vi "myCommOut_visa.vi"(0 "VISA资源名称":refnum<visa-resource-name>, 1 "freqs rows":i32[][](array[numeric]), 2 "log输入":string, 3 "默认幅值 Amp0":u8(ring)=2 items=["10.0", "5.0", "1.0", "0.5", "0.1", "0.05", "0.01"], 5 "实际幅值 Amp":u8(ring)=1 items=["= Amp0", "= Amp0 / freq"], 7 "t_wait":dbl=0.04, 9 "扰动注入模式":i32(ring) items=["无注入", "单相注入", "d轴注入", "q轴注入", "正(负)序注入"], 10 "最大同时扫频数":u32=5 min=1 max=10, 11 "错误输入（无错误）":errorcluster, 12 "基波频率":u32=50, 14 "存在DSP":bool) -> (4 "VISA资源名称 2":refnum<visa-resource-name>, 8 "error out":bool, 13 "log输出":string, 15 "错误输出":errorcluster)   [LabVIEW 2024]
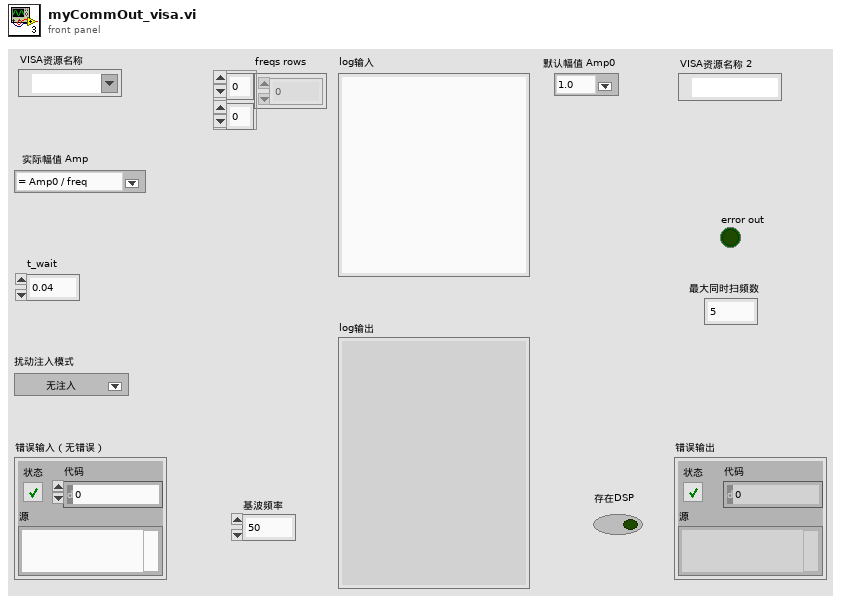
[diagram p1: front panel]
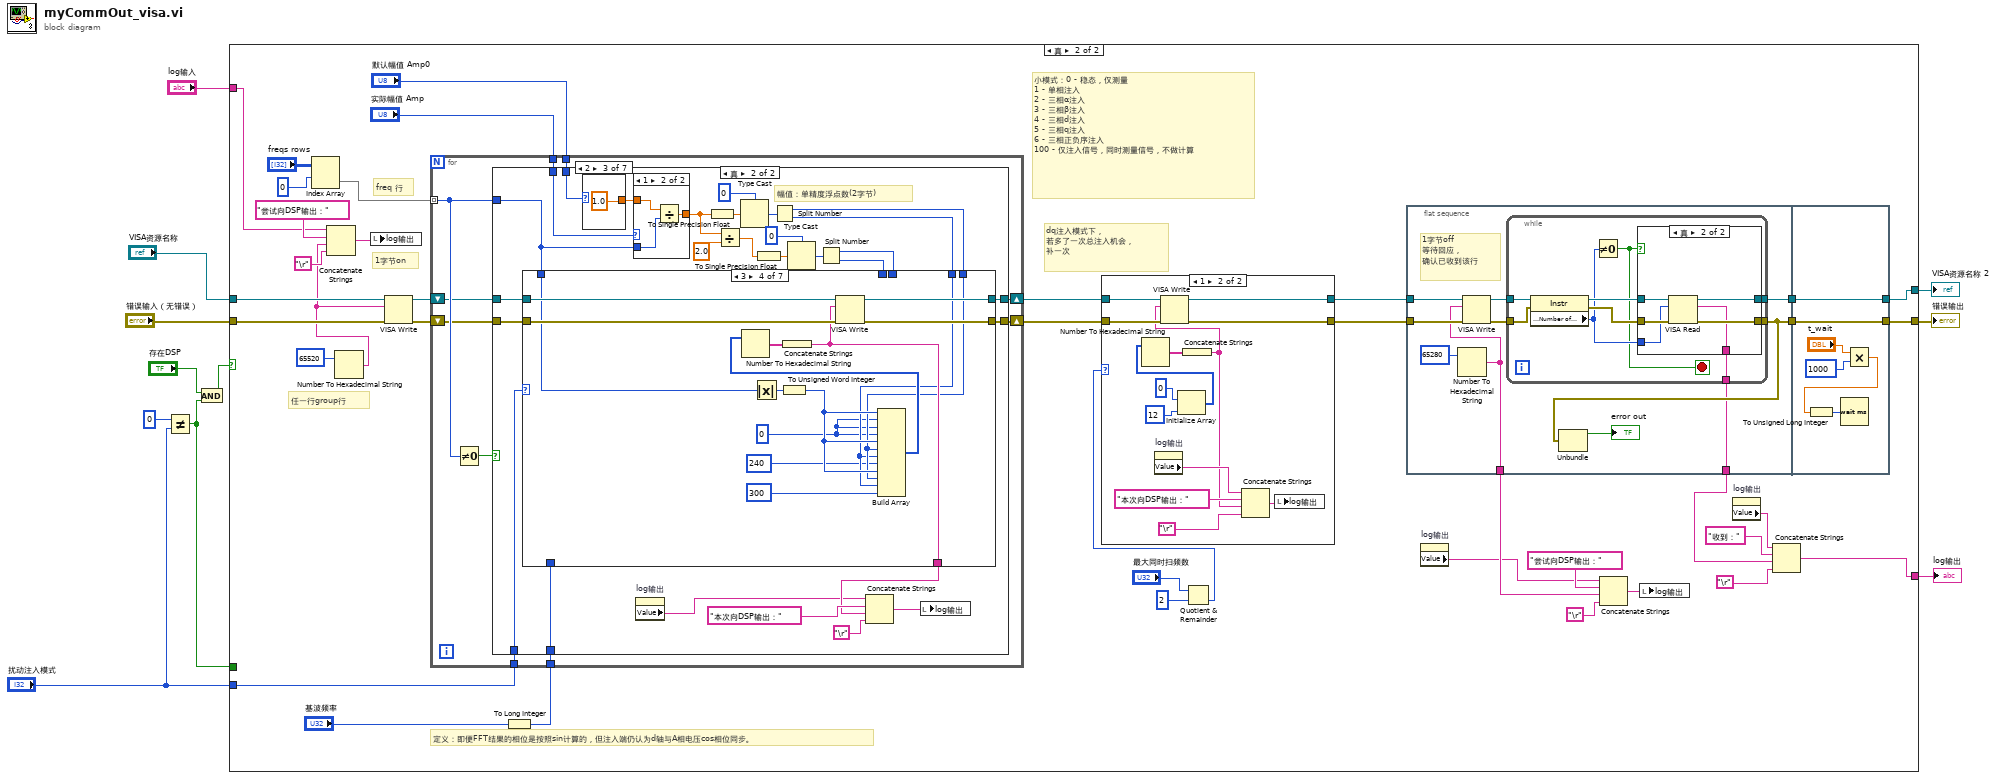
[diagram p0: block diagram]
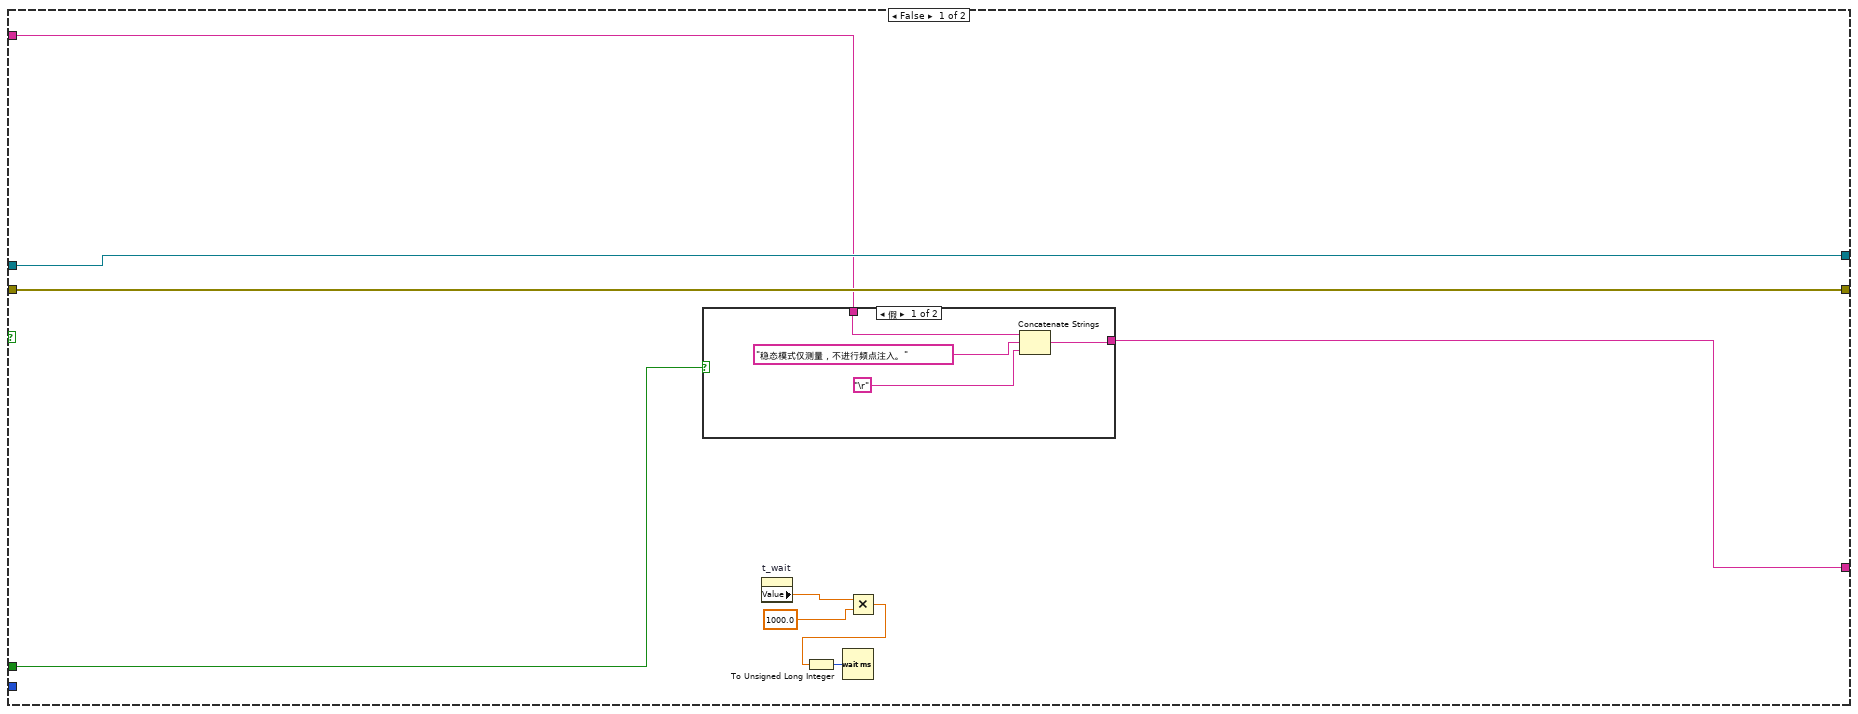
[diagram p2: hidden frame]
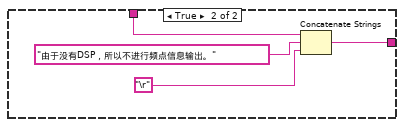
[diagram p3: hidden frame]
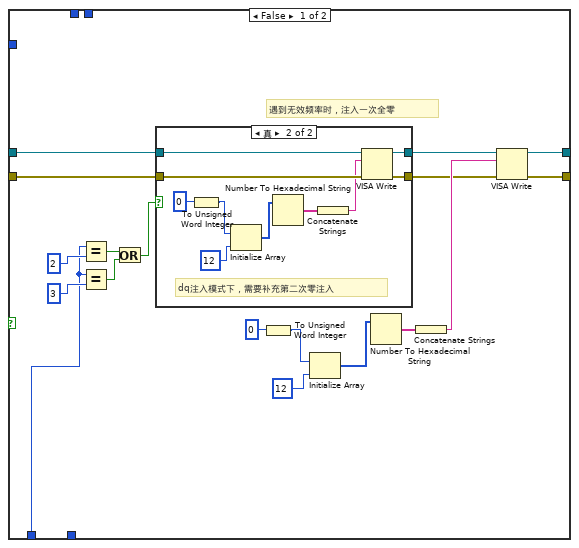
[diagram p6: hidden frame]
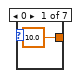
[diagram p9: hidden frame]
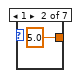
[diagram p10: hidden frame]
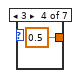
[diagram p11: hidden frame]
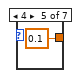
[diagram p12: hidden frame]
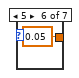
[diagram p13: hidden frame]
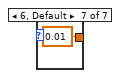
[diagram p14: hidden frame]
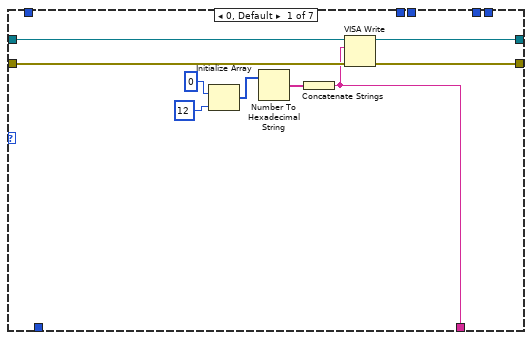
[diagram p15: hidden frame]
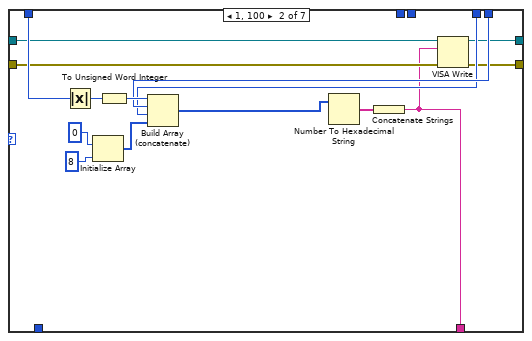
[diagram p16: hidden frame]
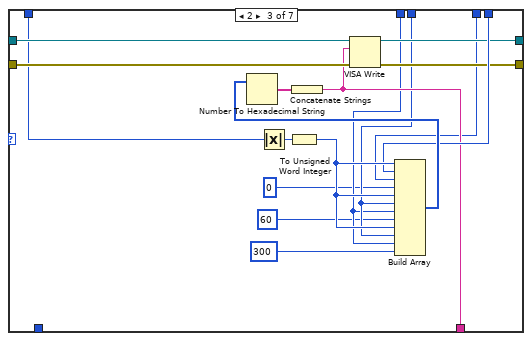
[diagram p17: hidden frame]
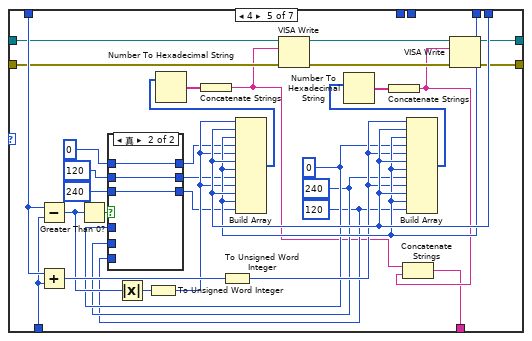
[diagram p18: hidden frame]
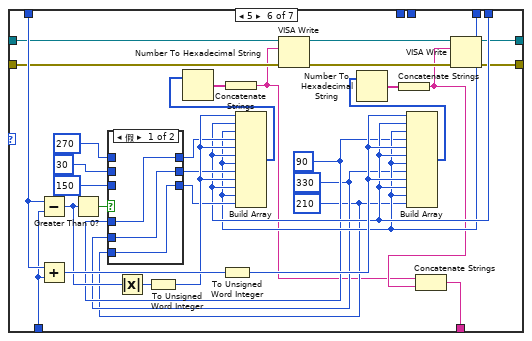
[diagram p20: hidden frame]
diagram:
  n1 = Not Equal?(x=0, y="扰动注入模式") -> (x != y?=w3:bool)
  n2 = And(x="存在DSP", y=w3) -> (x .and. y?=w4:bool)
  n3 = case shown="真" w4 {
    tunnel: "VISA资源名称" -> [w20 w54]
    tunnel: "错误输入（无错误）" -> [w19 w53]
    tunnel: [w20 w49] -> w9
    tunnel: [w19 w48] -> w8
    tunnel: "log输入" -> [w15 w43]
    tunnel: [w14 w38] -> w6
    tunnel: "扰动注入模式" -> [_ w29]
    tunnel: w3 -> [w12 _]
    frame False {
      n4 = case shown="假" w12 {
        tunnel: w15 -> [w21 w26]
        tunnel: [w22 w25] -> w14
        frame False {
          n5 = Concatenate Strings(w21, "稳态模式仅测量，不进行频点注入。", "\r") -> (w22:string)
        }
        frame True {
          n6 = Concatenate Strings(w26, "由于没有DSP，所以不进行频点信息输出。", "\r") -> (w25:string)
        }
      }
      n7 = property on="t_wait" class="DigNum (严格)"() -> ("Value"=w13:dbl)  [unwired: 2 in, 2 out]
      n8 = Multiply(x=w13, y=1000.0) -> (x*y=w18:dbl)
      n9 = To Unsigned Long Integer(number=w18) -> (unsigned 32bit integer=w17:u32)
      n10 = Wait (ms)(milliseconds to wait=w17) -> ()  [unwired: 1 out]
    }
    frame True {
      # "小模式：0 - 稳态，仅测量\n1 - 单相注入\n2 - 三相α注入\n3 - 三相β注入\n4 - 三相d注入\n5 - 三相q注入\n6 - 三相正负序注入\n100 - 仅注入信号，同时测量信号，不做计算"
      # "freq 行"
      # "dq注入模式下，\n若多了一次总注入机会，\n补一次"
      # "任一行group行"
      # "1字节on"
      # "定义：即便FFT结果的相位是按照sin计算的，但注入端仍认为d轴与A相电压cos相位同步。"
      n11 = Index Array(array="freqs rows", index (row)=0 ("索引")) -> (element=w31:i32[])  [unwired: 1 in]
      n12 = Number To Hexadecimal String(2:u16 65520) -> (0:w45:string)  [unwired: 1 in]
      n13 = Concatenate Strings(w43, "尝试向DSP输出：", w45, "\r") -> (w44:string)
      n14 = local write "log输出"(w44) -> ()
      n15 = VISA Write(VISA resource name=w54, write buffer=w45, error in (no error)=w53) -> (VISA resource name out=w62:refnum<visa-resource-name>, error out=w63:errorcluster)  [unwired: 1 out]
      n16 = To Long Integer(number="基波频率") -> (32bit integer=w55:i32)
      n17 = for {
        shift-right: [w121] -> w60
        shift-left: w62 -> [w123]
        shift-right: [w120] -> w59
        shift-left: w63 -> [w122]
        tunnel: w31 -> [w125] mode=indexing
        tunnel: w29 -> [w119]
        tunnel: "实际幅值 Amp" -> [w118]
        tunnel: "默认幅值 Amp0" -> [w117]
        tunnel: w55 -> [w116]
        n18 = Not Equal To 0?(x=w125) -> (x != 0?=w124:bool)
        n19 = case shown="真" w124 {
          tunnel: w125 -> [_ w169]
          tunnel: [w127 w174] -> w120
          tunnel: w123 -> [w139 w177]
          tunnel: [w128 w175] -> w121
          tunnel: w122 -> [w140 w176]
          tunnel: w119 -> [w133 w173]
          tunnel: w118 -> [_ w172]
          tunnel: w117 -> [_ w171]
          tunnel: w116 -> [_ w170]
          frame False {
            # "遇到无效频率时，注入一次全零"
            n20 = Equal?(x=w133, y=2) -> (x = y?=w135:bool)
            n21 = Equal?(x=w133, y=3) -> (x = y?=w136:bool)
            n22 = Or(x=w135, y=w136) -> (x .or. y?=w134:bool)
            n23 = case shown="真" w134 {
              tunnel: w140 -> [w144 w151]
              tunnel: w139 -> [w145 w152]
              tunnel: [w145 w146] -> w129
              tunnel: [w144 w147] -> w126
              frame False {
              }
              frame True {
                # "dq注入模式下，需要补充第二次零注入"
                n24 = To Unsigned Word Integer(number=u16 0) -> (unsigned 16bit integer=w154:u16)
                n25 = Initialize Array(w154, 12 ("维数大小")) -> (w149:u16[])
                n26 = Number To Hexadecimal String(2:w149) -> (0:w150:string[])  [unwired: 1 in]
                n27 = Concatenate Strings(w150) -> (w148:string)
                n28 = VISA Write(VISA resource name=w152, write buffer=w148, error in (no error)=w151) -> (VISA resource name out=w146:refnum<visa-resource-name>, error out=w147:errorcluster)  [unwired: 1 out]
              }
            }
            n29 = To Unsigned Word Integer(number=u16 0) -> (unsigned 16bit integer=w142:u16)
            n30 = Initialize Array(w142, 12 ("维数大小")) -> (w131:u16[])
            n31 = Number To Hexadecimal String(2:w131) -> (0:w132:string[])  [unwired: 1 in]
            n32 = Concatenate Strings(w132) -> (w130:string)
            n33 = VISA Write(VISA resource name=w129, write buffer=w130, error in (no error)=w126) -> (VISA resource name out=w128:refnum<visa-resource-name>, error out=w127:errorcluster)  [unwired: 1 out]
          }
          frame True {
            # "幅值：单精度浮点数(2字节)"
            n34 = case shown="2" w171 {
              tunnel: [10.0 5.0 1.0 0.5 0.1 0.05 0.01] -> w183
              frame 0 {
              }
              frame 1 {
              }
              frame 2 {
              }
              frame 3 {
              }
              frame 4 {
              }
              frame 5 {
              }
              frame 6, Default {
              }
            }
            n35 = case shown="1" w172 {
              tunnel: w183 -> [w184 w187]
              tunnel: w169 -> [_ w186]
              tunnel: [w184 w185] -> w163
              frame 0, Default {
              }
              frame 1 {
                n36 = Divide(x=w187, y=w186) -> (x/y=w185:dbl)
              }
            }
            n37 = property on="log输出" class="Str"() -> ("Value"=w165:string)  [unwired: 2 in, 2 out]
            n38 = To Single Precision Float(number=w163) -> (single precision float=w182:sgl)
            n39 = Divide(x=w163, y=2.0) -> (x/y=w159:dbl)
            n40 = Type Cast(type=0, x=w182) -> (*(type *) &x=w180:i32)
            n41 = To Single Precision Float(number=w159) -> (single precision float=w161:sgl)
            n42 = Split Number(x=w180) -> (hi(x)=w179:u16, lo(x)=w178:u16)
            n43 = Type Cast(type=0, x=w161) -> (*(type *) &x=w156:i32)
            n44 = Split Number(x=w156) -> (hi(x)=w158:u16, lo(x)=w157:u16)
            n45 = case shown="3" w173 {
              tunnel: w169 -> [_ w217 w228 w244 w279 w311 w340]
              tunnel: w179 -> [_ w213 w229 w240 w281 w310 w339]
              tunnel: w178 -> [_ w212 w224 w239 w280 w309 w338]
              tunnel: [w200 w209 w225 w241 w257 w296 w332] -> w175
              tunnel: w177 -> [w197 w210 w231 w246 w262 w298 w335]
              tunnel: [w199 w207 w226 w242 w258 w295 w333] -> w174
              tunnel: w176 -> [w198 w208 w230 w245 w261 w297 w334]
              tunnel: w170 -> [_ _ _ _ w264 w302 _]
              tunnel: [w195 w204 w227 w243 w251 w289 w330] -> w166
              tunnel: w158 -> [_ _ w223 _ _ _ _]
              tunnel: w157 -> [_ _ w222 _ _ _ _]
              frame 0, Default {
                n46 = Initialize Array(u16 0, 12 ("维数大小")) -> (w196:u16[])
                n47 = Number To Hexadecimal String(2:w196) -> (0:w201:string[])  [unwired: 1 in]
                n48 = Concatenate Strings(w201) -> (w195:string)
                n49 = VISA Write(VISA resource name=w197, write buffer=w195, error in (no error)=w198) -> (VISA resource name out=w200:refnum<visa-resource-name>, error out=w199:errorcluster)  [unwired: 1 out]
              }
              frame 1, 100 {
                n50 = Absolute Value(x=w217) -> (abs(x)=w218:i32)
                n51 = Initialize Array(u16 0, 8 ("维数大小")) -> (w206:u16[])
                n52 = To Unsigned Word Integer(number=w218) -> (unsigned 16bit integer=w214:u16)
                n53 = Build Array (concatenate)(w214, w213, w212, w206) -> (w205:u16[])
                n54 = Number To Hexadecimal String(2:w205) -> (0:w211:string[])  [unwired: 1 in]
                n55 = Concatenate Strings(w211) -> (w204:string)
                n56 = VISA Write(VISA resource name=w210, write buffer=w204, error in (no error)=w208) -> (VISA resource name out=w209:refnum<visa-resource-name>, error out=w207:errorcluster)  [unwired: 1 out]
              }
              frame 2 {
                n57 = Absolute Value(x=w228) -> (abs(x)=w235:i32)
                n58 = To Unsigned Word Integer(number=w235) -> (unsigned 16bit integer=w234:u16)
                n59 = Build Array(w234, w229, w224, u16 0, w234, w223, w222, u16 60, w234, w223, w222, u16 300) -> (w232:u16[])
                n60 = Number To Hexadecimal String(2:w232) -> (0:w233:string[])  [unwired: 1 in]
                n61 = Concatenate Strings(w233) -> (w227:string)
                n62 = VISA Write(VISA resource name=w231, write buffer=w227, error in (no error)=w230) -> (VISA resource name out=w225:refnum<visa-resource-name>, error out=w226:errorcluster)  [unwired: 1 out]
              }
              frame 3 {
                w238 = u16 0
                n63 = Absolute Value(x=w244) -> (abs(x)=w250:i32)
                n64 = To Unsigned Word Integer(number=w250) -> (unsigned 16bit integer=w249:u16)
                n65 = Build Array(w249, w238, w238, w238, w249, w240, w239, u16 240, w249, w240, w239, u16 300) -> (w247:u16[])
                n66 = Number To Hexadecimal String(2:w247) -> (0:w248:string[])  [unwired: 1 in]
                n67 = Concatenate Strings(w248) -> (w243:string)
                n68 = VISA Write(VISA resource name=w246, write buffer=w243, error in (no error)=w245) -> (VISA resource name out=w241:refnum<visa-resource-name>, error out=w242:errorcluster)  [unwired: 1 out]
              }
              frame 4 {
                w265 = u16 120
                w266 = u16 240
                w267 = u16 0
                n69 = Subtract(x=w279, y=w264) -> (x-y=w276:i32)
                n70 = Add(x=w279, y=w264) -> (x+y=w278:i32)
                n71 = Greater Than 0?(x=w276) -> (x > 0?=w274:bool)
                n72 = case shown="真" w274 {
                  tunnel: u16 0 -> [_ w288]
                  tunnel: u16 120 -> [_ w287]
                  tunnel: u16 240 -> [_ w286]
                  tunnel: [w283 w288] -> w270
                  tunnel: [w284 w287] -> w269
                  tunnel: [w285 w286] -> w268
                  tunnel: w267 -> [w283 _]
                  tunnel: w266 -> [w284 _]
                  tunnel: w265 -> [w285 _]
                  frame False {
                  }
                  frame True {
                  }
                }
                n73 = Absolute Value(x=w276) -> (abs(x)=w282:i32)
                n74 = To Unsigned Word Integer(number=w282) -> (unsigned 16bit integer=w275:u16)
                n75 = To Unsigned Word Integer(number=w278) -> (unsigned 16bit integer=w277:u16)
                n76 = Build Array(w275, w281, w280, w270, w275, w281, w280, w269, w275, w281, w280, w268) -> (w254:u16[])
                n77 = Number To Hexadecimal String(2:w254) -> (0:w255:string[])  [unwired: 1 in]
                n78 = Concatenate Strings(w255) -> (w253:string)
                n79 = VISA Write(VISA resource name=w262, write buffer=w253, error in (no error)=w261) -> (VISA resource name out=w260:refnum<visa-resource-name>, error out=w259:errorcluster)  [unwired: 1 out]
                n80 = Build Array(w277, w281, w280, w267, w277, w281, w280, w266, w277, w281, w280, w265) -> (w256:u16[])
                n81 = Number To Hexadecimal String(2:w256) -> (0:w263:string[])  [unwired: 1 in]
                n82 = Concatenate Strings(w263) -> (w252:string)
                n83 = Concatenate Strings(w253, w252) -> (w251:string)
                n84 = VISA Write(VISA resource name=w260, write buffer=w252, error in (no error)=w259) -> (VISA resource name out=w257:refnum<visa-resource-name>, error out=w258:errorcluster)  [unwired: 1 out]
              }
              frame 5 {
                w306 = u16 210
                w307 = u16 330
                w308 = u16 90
                n85 = Subtract(x=w311, y=w302) -> (x-y=w317:i32)
                n86 = Add(x=w311, y=w302) -> (x+y=w319:i32)
                n87 = Greater Than 0?(x=w317) -> (x > 0?=w315:bool)
                n88 = case shown="假" w315 {
                  tunnel: u16 270 -> [_ w326]
                  tunnel: u16 30 -> [_ w325]
                  tunnel: u16 150 -> [_ w324]
                  tunnel: [w321 w326] -> w314
                  tunnel: [w322 w325] -> w313
                  tunnel: [w323 w324] -> w312
                  tunnel: w308 -> [w321 _]
                  tunnel: w307 -> [w322 _]
                  tunnel: w306 -> [w323 _]
                  frame False {
                  }
                  frame True {
                  }
                }
                n89 = Absolute Value(x=w317) -> (abs(x)=w320:i32)
                n90 = To Unsigned Word Integer(number=w320) -> (unsigned 16bit integer=w316:u16)
                n91 = To Unsigned Word Integer(number=w319) -> (unsigned 16bit integer=w318:u16)
                n92 = Build Array(w316, w310, w309, w314, w316, w310, w309, w313, w316, w310, w309, w312) -> (w292:u16[])
                n93 = Number To Hexadecimal String(2:w292) -> (0:w293:string[])  [unwired: 1 in]
                n94 = Concatenate Strings(w293) -> (w290:string)
                n95 = VISA Write(VISA resource name=w298, write buffer=w290, error in (no error)=w297) -> (VISA resource name out=w299:refnum<visa-resource-name>, error out=w300:errorcluster)  [unwired: 1 out]
                n96 = Build Array(w318, w310, w309, w308, w318, w310, w309, w307, w318, w310, w309, w306) -> (w294:u16[])
                n97 = Number To Hexadecimal String(2:w294) -> (0:w301:string[])  [unwired: 1 in]
                n98 = Concatenate Strings(w301) -> (w291:string)
                n99 = Concatenate Strings(w290, w291) -> (w289:string)
                n100 = VISA Write(VISA resource name=w299, write buffer=w291, error in (no error)=w300) -> (VISA resource name out=w296:refnum<visa-resource-name>, error out=w295:errorcluster)  [unwired: 1 out]
              }
              frame 6 {
                n101 = Greater Than 0?(x=w340) -> (x > 0?=w343:bool)
                n102 = case shown="真" w343 {
                  tunnel: [w345 w348] -> w329
                  tunnel: u16 240 -> [w346 w348]
                  tunnel: [w346 w347] -> w327
                  tunnel: u16 120 -> [w345 w347]
                  frame False {
                  }
                  frame True {
                  }
                }
                n103 = Absolute Value(x=w340) -> (abs(x)=w344:i32)
                n104 = To Unsigned Word Integer(number=w344) -> (unsigned 16bit integer=w337:u16)
                n105 = Build Array(w337, w339, w338, u16 0, w337, w339, w338, w329, w337, w339, w338, w327) -> (w331:u16[])
                n106 = Number To Hexadecimal String(2:w331) -> (0:w336:string[])  [unwired: 1 in]
                n107 = Concatenate Strings(w336) -> (w330:string)
                n108 = VISA Write(VISA resource name=w335, write buffer=w330, error in (no error)=w334) -> (VISA resource name out=w332:refnum<visa-resource-name>, error out=w333:errorcluster)  [unwired: 1 out]
              }
            }
            n109 = Concatenate Strings(w165, "本次向DSP输出：", w166, "\r") -> (w164:string)
            n110 = local write "log输出"(w164) -> ()
          }
        }
      }
      n111 = Quotient & Remainder(x="最大同时扫频数", y=u32 2) -> (floor(x/y)=w56:u32)  [unwired: 1 out]
      n112 = case shown="1" w56 {
        tunnel: [w102 w110] -> w58
        tunnel: w60 -> [w102 w111]
        tunnel: [w101 w109] -> w57
        tunnel: w59 -> [w101 w108]
        frame 0, Default {
        }
        frame 1 {
          n113 = property on="log输出" class="Str"() -> ("Value"=w107:string)  [unwired: 2 in, 2 out]
          n114 = Initialize Array(u16 0, 12 ("维数大小")) -> (w112:u16[])
          n115 = Number To Hexadecimal String(2:w112) -> (0:w113:string[])  [unwired: 1 in]
          n116 = Concatenate Strings(w113) -> (w103:string)
          n117 = VISA Write(VISA resource name=w111, write buffer=w103, error in (no error)=w108) -> (VISA resource name out=w110:refnum<visa-resource-name>, error out=w109:errorcluster)  [unwired: 1 out]
          n118 = Concatenate Strings(w107, "本次向DSP输出：", w103, "\r") -> (w106:string)
          n119 = local write "log输出"(w106) -> ()
        }
      }
      n120 = flat-sequence {
        tunnel: w58 -> [w76]
        tunnel: w57 -> [w75]
        tunnel: [w72] -> w67
        tunnel: [w71] -> w66
        tunnel: [w69] -> w37
        tunnel: [w68] -> w36
        tunnel: [w99] -> w48
        tunnel: [w100] -> w49
        tunnel: w67 -> [w100]
        tunnel: w66 -> [w99]
        frame #0 {
          # "1字节off\n等待回应，\n确认已收到该行"
          n121 = Number To Hexadecimal String(2:u16 65280) -> (0:w68:string)  [unwired: 1 in]
          n122 = VISA Write(VISA resource name=w76, write buffer=w68, error in (no error)=w75) -> (VISA resource name out=w74:refnum<visa-resource-name>, error out=w73:errorcluster)  [unwired: 1 out]
          n123 = while {
            tunnel: [w82] -> w71
            tunnel: [w81] -> w72
            tunnel: w74 -> [w80]
            tunnel: w73 -> [w79]
            tunnel: [w78] -> w69
            stop <- w83 stop-if-true
            n124 = property class="Instr"(reference=w80, error in=w79) -> (reference out=w86:refnum<visa-resource-name>, error out=w85:errorcluster, "Serial Settings:Number of Bytes at Serial Port"=w84:u32)
            n125 = Not Equal To 0?(x=w84) -> (x != 0?=w83:bool)
            n126 = case shown="真" w83 {
              tunnel: w86 -> [w88 w93]
              tunnel: w85 -> [w87 w94]
              tunnel: w84 -> [_ w92]
              tunnel: [w87 w91] -> w82
              tunnel: [w88 w90] -> w81
              tunnel: [_ w89] -> w78
              frame False {
              }
              frame True {
                n127 = VISA Read(VISA resource name=w93, byte count=w92, error in (no error)=w94) -> (VISA resource name out=w90:refnum<visa-resource-name>, read buffer=w89:string, error out=w91:errorcluster)  [unwired: 1 out]
              }
            }
          }
          n128 = Unbundle(w71) -> ("status"=→"error out":bool)  [unwired: 2 out]
        }
        frame #1 {
          n129 = Multiply(x="t_wait", y=1000) -> (x*y=w98:dbl)
          n130 = To Unsigned Long Integer(number=w98) -> (unsigned 32bit integer=w97:u32)
          n131 = Wait (ms)(milliseconds to wait=w97) -> ()  [unwired: 1 out]
        }
      }
      n132 = property on="log输出" class="Str"() -> ("Value"=w34:string)  [unwired: 2 in, 2 out]
      n133 = Concatenate Strings(w34, "尝试向DSP输出：", w36, "\r") -> (w33:string)
      n134 = local write "log输出"(w33) -> ()
      n135 = property on="log输出" class="Str"() -> ("Value"=w35:string)  [unwired: 2 in, 2 out]
      n136 = Concatenate Strings(w35, "收到：", w37, "\r") -> (w38:string)
    }
  }
  "错误输出" <- w8
  "VISA资源名称 2" <- w9
  "log输出" <- w6
